vi "VPA QC DAQ Loop.vi"(8 "error in (no error)":errorcluster, 10 "DAQ Ref Cluster":T2, 11 "DAQ Q":T1) -> (0 "error out":errorcluster)   [LabVIEW 2013]
uses:
  Controls/VPA QC DAQ Ref Cluster.ctl
  Controls/VPA QC Scale Communication Settings DVR.ctl
  Controls/VPA QC Scale Communication Settings.ctl
  Controls/VPA QC DAQ Q.ctl
  Controls/VPA QC DAQ Cmd Enum.ctl
  <vilib>/DAQmx/create/channels.llb/DAQmx Create Channel (AI-Voltage-Basic).vi
  <userlib>/_MGI/Timing/MGI Wait/MGI Wait (U32).vi
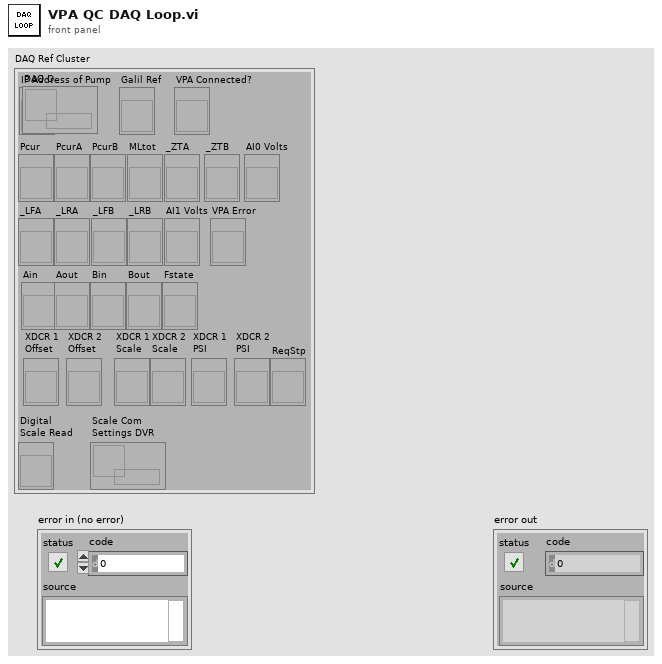
[diagram p1: front panel]
types:
  T1 = typedef "VPA QC DAQ Q.ctl" = refnum<queue>
  T2 = typedef "VPA QC DAQ Ref Cluster.ctl" = cluster{"IP Address of Pump":refnum<vi>, "Galil Ref":refnum<vi>, "VPA Connected?":refnum<vi>, "Pcur":refnum<vi>, "PcurA":refnum<vi>, "PcurB":refnum<vi>, "MLtot":refnum<vi>, "_LFA":refnum<vi>, "_LRA":refnum<vi>, "_LFB":refnum<vi>, "_LRB":refnum<vi>, "_ZTA":refnum<vi>, "_ZTB":refnum<vi>, "AI0 Volts":refnum<vi>, "AI1 Volts":refnum<vi>, "VPA Error":refnum<vi>, "Ain":refnum<vi>, "Aout":refnum<vi>, "Bin":refnum<vi>, "Bout":refnum<vi>, "Fstate":refnum<vi>, "XDCR 1\nOffset":refnum<vi>, "XDCR 2 \nOffset":refnum<vi>, "XDCR 1\nScale":refnum<vi>, "XDCR 2\nScale":refnum<vi>, "XDCR 1\nPSI":refnum<vi>, "XDCR 2\nPSI":refnum<vi>, "ReqStp":refnum<vi>, "Digital \nScale Read":refnum<vi>, "Scale Com\nSettings DVR":T3}
  T3 = typedef "VPA QC Scale Communication Settings DVR.ctl" = refnum<data-value>
  T4 = typedef "VPA QC DAQ Cmd Enum.ctl" = enum16{"Connect", "Disconnect", "Quit", "Close All Valves", "Burn Calibration", "E-Stop", "Set ZC1", "Set ZC0", "Set ZR", "Open Outlet Valves"}
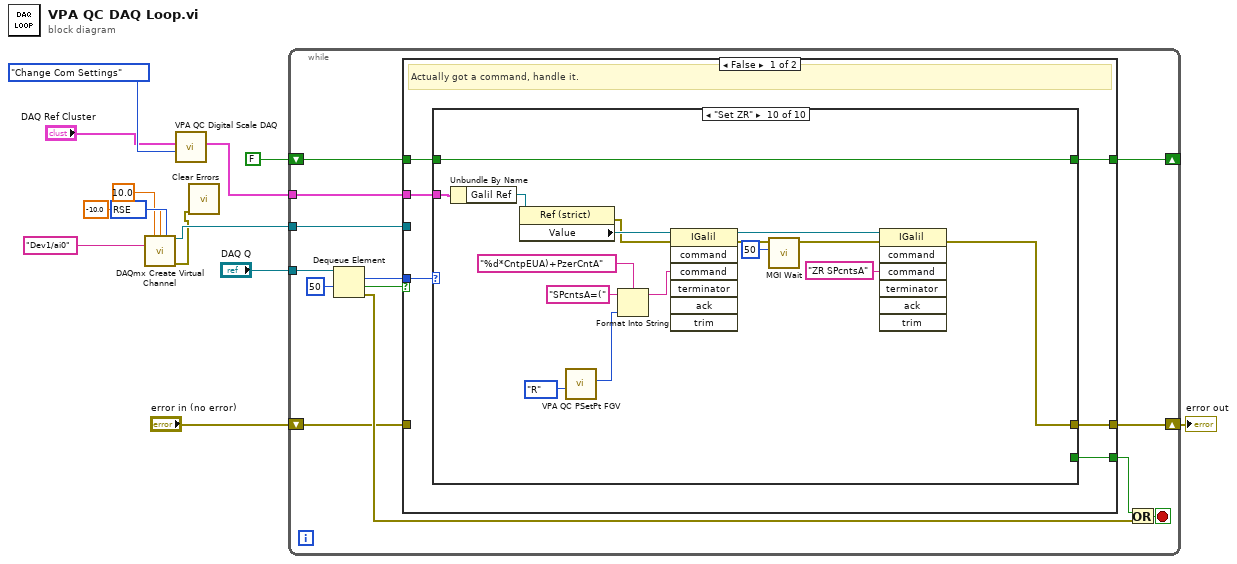
[diagram p0: block diagram]
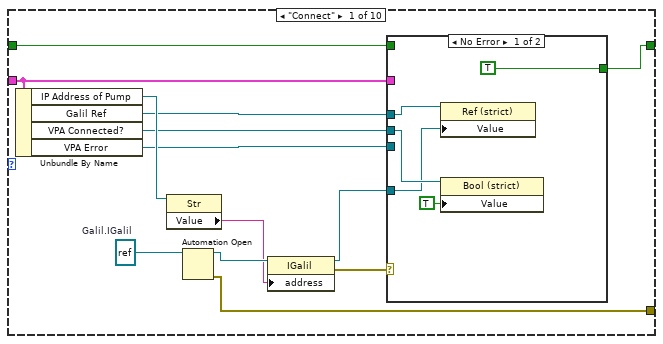
[diagram p2: hidden frame]
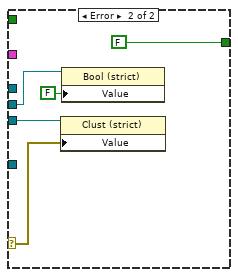
[diagram p3: hidden frame]
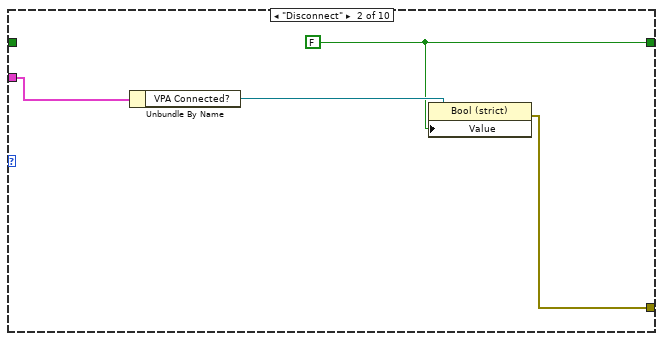
[diagram p4: hidden frame]
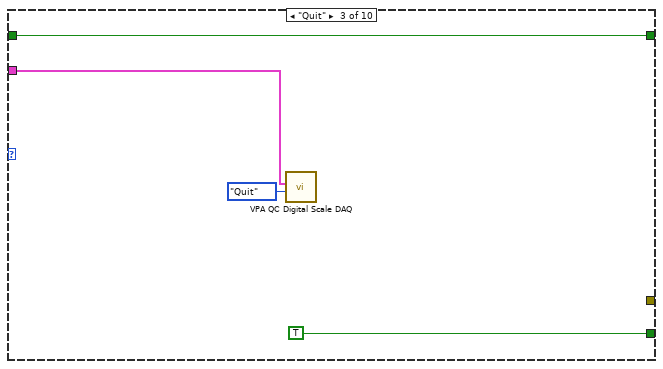
[diagram p5: hidden frame]
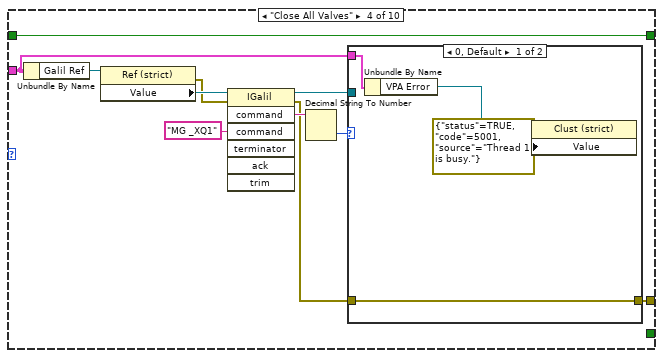
[diagram p6: hidden frame]
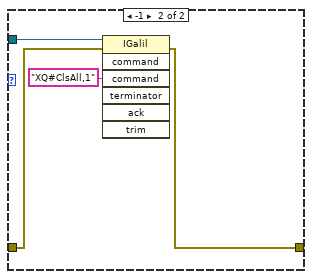
[diagram p7: hidden frame]
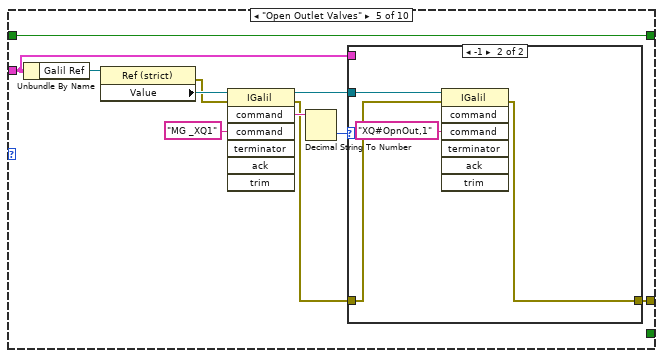
[diagram p8: hidden frame]
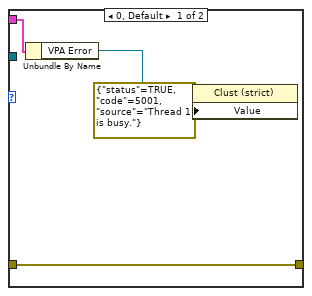
[diagram p9: hidden frame]
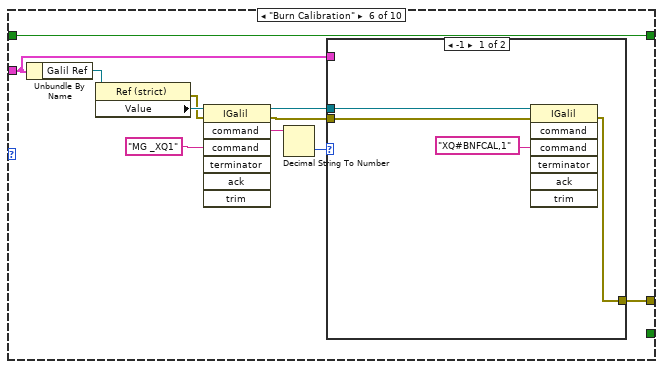
[diagram p10: hidden frame]
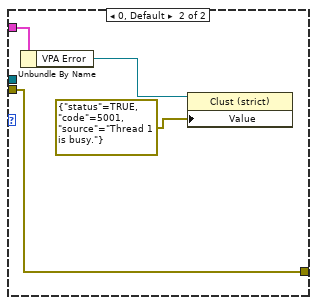
[diagram p11: hidden frame]
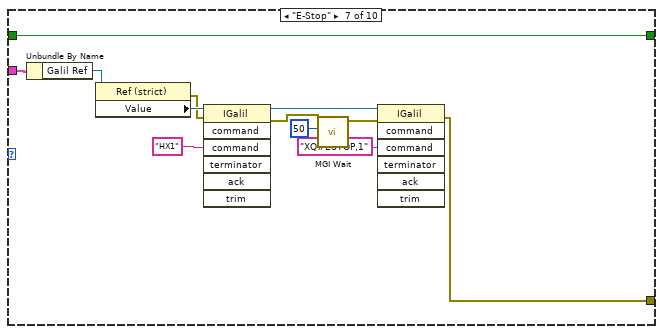
[diagram p12: hidden frame]
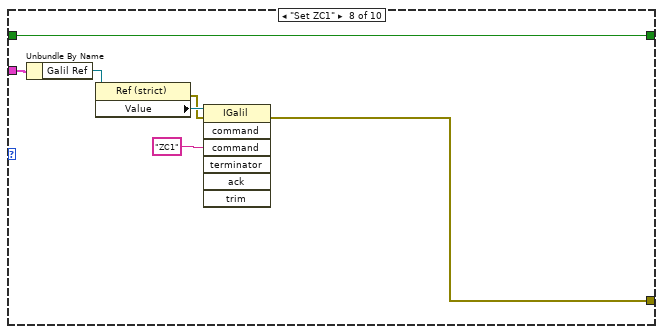
[diagram p13: hidden frame]
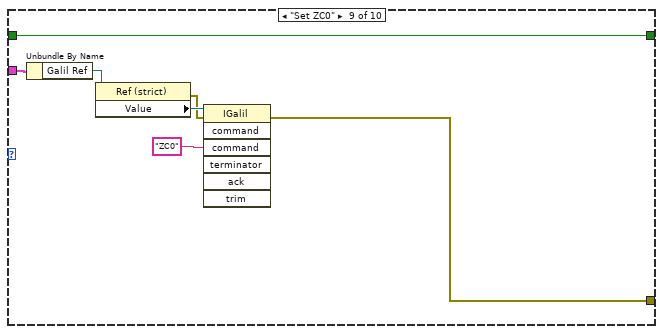
[diagram p14: hidden frame]
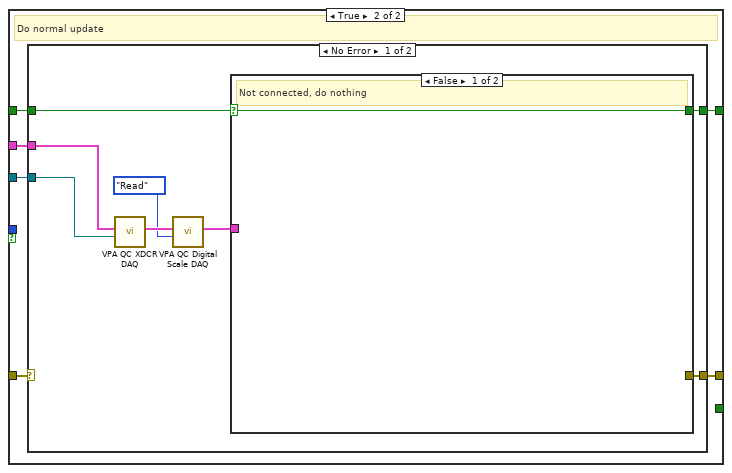
[diagram p15: hidden frame]
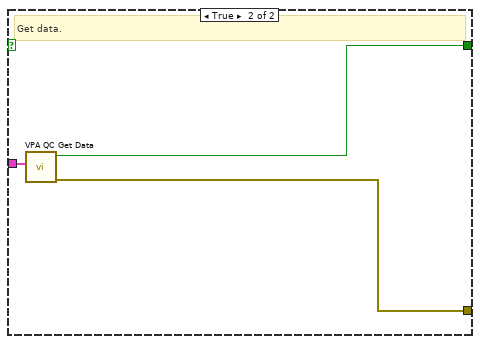
[diagram p16: hidden frame]
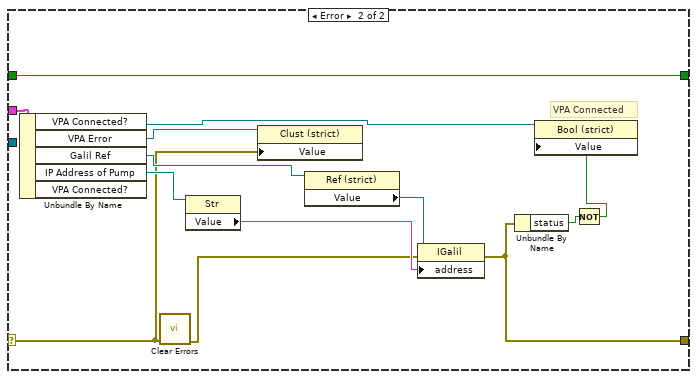
[diagram p17: hidden frame]
diagram:
  w8 = 10083 items=["default"=-1, "RSE"=10083, "NRSE"=10078, "Differential"=10106, "Pseudodifferential"=12529] ("input terminal configuration")
  n1 = call-poly <vilib>:"DAQmx Create Virtual Channel.vi"("maximum value"=10.0, "minimum value"=-10.0, "input terminal configuration"=w8, "physical channels"="Dev1/ai0") -> ("task out"=w9:refnum<k21>, "error out"=w1:errorcluster)  [unwired: 10 in]
  n2 = call "VPA QC Digital Scale DAQ.vi"("Function"=enum16{"Change Com Settings", "Read"}."Change Com Settings", "DAQ Ref Cluster"="DAQ Ref Cluster") -> ("DAQ Ref Cluster Out"=w2:T2)  [unwired: 9 in]
  n3 = call <vilib>:"Clear Errors.vi"("error in (no error)"=w1) -> ()  [unwired: 6 in, 1 out]
  n4 = while {
    tunnel: w2 -> [w22]
    tunnel: "DAQ Q" -> [w25]
    shift-right: [w19] -> w11
    shift-left: "error in (no error)" -> [w14]
    shift-right: [w20] -> _
    shift-left: FALSE -> [w21]
    tunnel: w9 -> [w18]
    stop <- w15 stop-if-true
    n5 = Dequeue Element(queue=w25, timeout in ms (-1)=50) -> (element=w24:T4, timed out?=w23:bool, error out=w17:errorcluster)  [unwired: 1 in, 1 out]
    n6 = case shown="False" w23 {
      tunnel: w24 -> [w32 _]
      tunnel: [w31 _] -> w16
      tunnel: w14 -> [_ w163]
      tunnel: w22 -> [w28 w164]
      tunnel: w21 -> [w30 w168]
      tunnel: [w29 w167] -> w20
      tunnel: [w27 w166] -> w19
      tunnel: w18 -> [_ w165]
      frame False {
        # "Actually got a command, handle it."
        n7 = case shown="\"Set ZR\"" w32 {
          tunnel: [_ _ TRUE _ _ _ _ _ _ _] -> w31
          tunnel: w30 -> [w41 _ w62 w74 w93 w112 w132 w139 w146 w162]
          tunnel: [w35 w57 w62 w74 w93 w112 w132 w139 w146 w162] -> w29
          tunnel: w28 -> [w39 w59 w61 w65 w84 w105 w128 w135 w142 w159]
          tunnel: [w33 w56 _ w66 w85 w102 w121 w133 w140 w149] -> w27
          frame "Connect" {
            w45 = refnum<k7> refnum  # Galil.IGalil
            n8 = Unbundle By Name(w39) -> ("IP Address of Pump"=w44:refnum<vi>, "Galil Ref"=w38:refnum<vi>, "VPA Connected?"=w37:refnum<vi>, "VPA Error"=w34:refnum<vi>)
            n9 = property class="Str"(reference=w44) -> ("Value"=w42:string)  [unwired: 1 in, 2 out]
            n10 = Automation Open(Automation Refnum=w45) -> (Automation Refnum=w43:refnum<k7>, error out=w33:errorcluster)  [unwired: 3 in]
            n11 = property class="IGalil"(reference=w43, "address"=w42) -> (reference out=w36:refnum<k7>, error out=w40:errorcluster)  [unwired: 1 in]
            n12 = case shown="No Error" w40 {
              selector: w40 -> [_ w53]
              tunnel: w41 -> [_ _]
              tunnel: w39 -> [_ _]
              tunnel: w38 -> [w50 _]
              tunnel: w37 -> [w49 w52]
              tunnel: w36 -> [w48 _]
              tunnel: [TRUE FALSE] -> w35
              tunnel: w34 -> [_ w54]
              frame No Error {
                n13 = property class="Ref (strict)"(reference=w50, "Value"=w48) -> ()  [unwired: 1 in, 2 out]
                n14 = property class="Bool (strict)"(reference=w49, "Value"=TRUE) -> ()  [unwired: 1 in, 2 out]
              }
              frame Error {
                n15 = property class="Clust (strict)"(reference=w54, "Value"=w53) -> ()  [unwired: 1 in, 2 out]
                n16 = property class="Bool (strict)"(reference=w52, "Value"=FALSE) -> ()  [unwired: 1 in, 2 out]
              }
            }
          }
          frame "Disconnect" {
            w57 = FALSE
            n17 = Unbundle By Name(w59) -> ("VPA Connected?"=w58:refnum<vi>)
            n18 = property class="Bool (strict)"(reference=w58, "Value"=w57) -> (error out=w56:errorcluster)  [unwired: 1 in, 1 out]
          }
          frame "Quit" {
            n19 = call "VPA QC Digital Scale DAQ.vi"("Function"=enum16{"Change Com Settings", "Read", "Quit"}."Quit", "DAQ Ref Cluster"=w61) -> ()  [unwired: 9 in, 1 out]
          }
          frame "Close All Valves" {
            n20 = Unbundle By Name(w65) -> ("Galil Ref"=w73:refnum<vi>)
            n21 = property class="Ref (strict)"(reference=w73) -> (error out=w68:errorcluster, "Value"=w72:refnum<k7>)  [unwired: 1 in, 1 out]
            n22 = invoke class="IGalil" method="command"(reference=w72, error in=w68, "command"="MG _XQ1") -> (reference out=w64:refnum<k7>, error out=w67:errorcluster, "command"=w70:string)  [unwired: 4 in, 4 out]
            n23 = Decimal String To Number(string=w70) -> (number=w69:i32)  [unwired: 2 in, 1 out]
            n24 = case shown="0, Default" w69 {
              tunnel: w67 -> [w78 w80]
              tunnel: [w78 w79] -> w66
              tunnel: w65 -> [w77 _]
              tunnel: w64 -> [_ w82]
              frame 0, Default {
                n25 = Unbundle By Name(w77) -> ("VPA Error"=w76:refnum<vi>)
                n26 = property class="Clust (strict)"(reference=w76, "Value"=errorcluster {"status"=TRUE, "code"=5001, "source"="Thread 1 is busy."}) -> ()  [unwired: 1 in, 2 out]
              }
              frame -1 {
                n27 = invoke class="IGalil" method="command"(reference=w82, error in=w80, "command"="XQ#ClsAll,1") -> (error out=w79:errorcluster)  [unwired: 4 in, 6 out]
              }
            }
          }
          frame "Open Outlet Valves" {
            n28 = Unbundle By Name(w84) -> ("Galil Ref"=w92:refnum<vi>)
            n29 = property class="Ref (strict)"(reference=w92) -> (error out=w87:errorcluster, "Value"=w91:refnum<k7>)  [unwired: 1 in, 1 out]
            n30 = invoke class="IGalil" method="command"(reference=w91, error in=w87, "command"="MG _XQ1") -> (reference out=w83:refnum<k7>, error out=w86:errorcluster, "command"=w89:string)  [unwired: 4 in, 4 out]
            n31 = Decimal String To Number(string=w89) -> (number=w88:i32)  [unwired: 2 in, 1 out]
            n32 = case shown="-1" w88 {
              tunnel: w86 -> [w97 w99]
              tunnel: [w97 w98] -> w85
              tunnel: w84 -> [w96 _]
              tunnel: w83 -> [_ w101]
              frame 0, Default {
                n33 = Unbundle By Name(w96) -> ("VPA Error"=w95:refnum<vi>)
                n34 = property class="Clust (strict)"(reference=w95, "Value"=errorcluster {"status"=TRUE, "code"=5001, "source"="Thread 1 is busy."}) -> ()  [unwired: 1 in, 2 out]
              }
              frame -1 {
                n35 = invoke class="IGalil" method="command"(reference=w101, error in=w99, "command"="XQ#OpnOut,1") -> (error out=w98:errorcluster)  [unwired: 4 in, 6 out]
              }
            }
          }
          frame "Burn Calibration" {
            n36 = Unbundle By Name(w105) -> ("Galil Ref"=w111:refnum<vi>)
            n37 = property class="Ref (strict)"(reference=w111) -> (error out=w104:errorcluster, "Value"=w110:refnum<k7>)  [unwired: 1 in, 1 out]
            n38 = invoke class="IGalil" method="command"(reference=w110, error in=w104, "command"="MG _XQ1") -> (reference out=w106:refnum<k7>, error out=w103:errorcluster, "command"=w108:string)  [unwired: 4 in, 4 out]
            n39 = Decimal String To Number(string=w108) -> (number=w107:i32)  [unwired: 2 in, 1 out]
            n40 = case shown="-1" w107 {
              tunnel: w106 -> [w116 _]
              tunnel: w105 -> [_ w119]
              tunnel: w103 -> [w114 w117]
              tunnel: [w113 w117] -> w102
              frame -1 {
                n41 = invoke class="IGalil" method="command"(reference=w116, error in=w114, "command"="XQ#BNFCAL,1") -> (error out=w113:errorcluster)  [unwired: 4 in, 6 out]
              }
              frame 0, Default {
                n42 = Unbundle By Name(w119) -> ("VPA Error"=w120:refnum<vi>)
                n43 = property class="Clust (strict)"(reference=w120, "Value"=errorcluster {"status"=TRUE, "code"=5001, "source"="Thread 1 is busy."}) -> ()  [unwired: 1 in, 2 out]
              }
            }
          }
          frame "E-Stop" {
            n44 = Unbundle By Name(w128) -> ("Galil Ref"=w131:refnum<vi>)
            n45 = property class="Ref (strict)"(reference=w131) -> (error out=w127:errorcluster, "Value"=w130:refnum<k7>)  [unwired: 1 in, 1 out]
            n46 = invoke class="IGalil" method="command"(reference=w130, error in=w127, "command"="HX1") -> (reference out=w124:refnum<k7>, error out=w125:errorcluster)  [unwired: 4 in, 5 out]
            n47 = call-poly <userlib>:"MGI Wait.vi"("ms"=u32 50, "Error In"=w125) -> ("Error Out"=w122:errorcluster)  [unwired: 5 in]
            n48 = invoke class="IGalil" method="command"(reference=w124, error in=w122, "command"="XQ#ESTOP,1") -> (error out=w121:errorcluster)  [unwired: 4 in, 6 out]
          }
          frame "Set ZC1" {
            n49 = Unbundle By Name(w135) -> ("Galil Ref"=w138:refnum<vi>)
            n50 = property class="Ref (strict)"(reference=w138) -> (error out=w134:errorcluster, "Value"=w137:refnum<k7>)  [unwired: 1 in, 1 out]
            n51 = invoke class="IGalil" method="command"(reference=w137, error in=w134, "command"="ZC1") -> (error out=w133:errorcluster)  [unwired: 4 in, 6 out]
          }
          frame "Set ZC0" {
            n52 = Unbundle By Name(w142) -> ("Galil Ref"=w145:refnum<vi>)
            n53 = property class="Ref (strict)"(reference=w145) -> (error out=w141:errorcluster, "Value"=w144:refnum<k7>)  [unwired: 1 in, 1 out]
            n54 = invoke class="IGalil" method="command"(reference=w144, error in=w141, "command"="ZC0") -> (error out=w140:errorcluster)  [unwired: 4 in, 6 out]
          }
          frame "Set ZR" {
            n55 = Unbundle By Name(w159) -> ("Galil Ref"=w161:refnum<vi>)
            n56 = property class="Ref (strict)"(reference=w161) -> (error out=w158:errorcluster, "Value"=w160:refnum<k7>)  [unwired: 1 in, 1 out]
            n57 = call "VPA QC PSetPt FGV.vi"("Function"=enum16{"R", "W"}."R") -> ("PSetPt Out"=w155:u32)  [unwired: 9 in, 1 out]
            n58 = Format Into String(format string="%d*CntpEUA)+PzerCntA", initial string="SPcntsA=(", w155) -> (resulting string=w153:string)  [unwired: 1 in, 1 out]
            n59 = invoke class="IGalil" method="command"(reference=w160, error in=w158, "command"=w153) -> (reference out=w148:refnum<k7>, error out=w157:errorcluster)  [unwired: 4 in, 5 out]
            n60 = call-poly <userlib>:"MGI Wait.vi"("ms"=u32 50, "Error In"=w157) -> ("Error Out"=w150:errorcluster)  [unwired: 5 in]
            n61 = invoke class="IGalil" method="command"(reference=w148, error in=w150, "command"="ZR SPcntsA") -> (error out=w149:errorcluster)  [unwired: 4 in, 6 out]
          }
        }
      }
      frame True {
        # "Do normal update"
        n62 = case shown="No Error" w163 {
          selector: w163 -> [_ w183]
          tunnel: w168 -> [w176 w184]
          tunnel: [w175 w184] -> w167
          tunnel: [w174 w182] -> w166
          tunnel: w165 -> [w173 _]
          tunnel: w164 -> [w172 w181]
          frame No Error {
            n63 = call "VPA QC XDCR DAQ.vi"("task/channels in"=w173, "DAQ Ref Cluster"=w172) -> ("DAQ Ref Cluster Out"=w171:T2)  [unwired: 8 in, 1 out]
            n64 = call "VPA QC Digital Scale DAQ.vi"("Function"=enum16{"Change Com Settings", "Read"}."Read", "DAQ Ref Cluster"=w171) -> ("DAQ Ref Cluster Out"=w170:T2)  [unwired: 9 in]
            n65 = case shown="False" w176 {
              selector: w176 -> [w177 _]
              tunnel: [w177 w180] -> w175
              tunnel: [_ w178] -> w174
              tunnel: w170 -> [_ w179]
              frame False {
                # "Not connected, do nothing"
              }
              frame True {
                # "Get data."
                n66 = call "VPA QC Get Data.vi"("DAQ Ref Cluster"=w179) -> ("error out"=w178:errorcluster, "IP Connected?"=w180:bool)  [unwired: 9 in]
              }
            }
          }
          frame Error {
            # "VPA Connected"
            n67 = Unbundle By Name(w181) -> ("VPA Connected?"=w186:refnum<vi>, "VPA Error"=w193:refnum<vi>, "Galil Ref"=w191:refnum<vi>, "IP Address of Pump"=w192:refnum<vi>)  [unwired: 1 out]
            n68 = call <vilib>:"Clear Errors.vi"("error in (no error)"=w183) -> ("error out"=w188:errorcluster)  [unwired: 6 in]
            n69 = property class="Str"(reference=w192) -> ("Value"=w189:string)  [unwired: 1 in, 2 out]
            n70 = property class="Clust (strict)"(reference=w193, "Value"=w183) -> ()  [unwired: 1 in, 2 out]
            n71 = property class="Ref (strict)"(reference=w191) -> ("Value"=w190:refnum<k7>)  [unwired: 1 in, 2 out]
            n72 = property class="IGalil"(reference=w190, error in=w188, "address"=w189) -> (error out=w182:errorcluster)  [unwired: 1 out]
            n73 = Unbundle By Name(w182) -> ("status"=w187:bool)
            n74 = Not(x=w187) -> (.not. x?=w185:bool)
            n75 = property class="Bool (strict)"(reference=w186, "Value"=w185) -> ()  [unwired: 1 in, 2 out]
          }
        }
      }
    }
    n76 = Or(x=w16, y=w17) -> (x .or. y?=w15:bool)
  }
  "error out" <- w11
